vi "ParamsEntreferro.vi"(2 "paramsIn":variant=variant(cluster{"Componentes":cluster{"Pólo:":u16, "Amplitude:":dbl}[], "Num Polos":u16, "Folga Nominal":dbl, "Ruido":dbl} {"Componentes"=[], "Num Polos"=84, "Folga Nominal"=10.0, "Ruido"=1.0})) -> (16 "paramsOut":variant=variant(cluster{"Componentes":cluster{"Pólo:":u16, "Amplitude:":dbl}[], "Num Polos":u16, "Folga Nominal":dbl, "Ruido":dbl} {"Componentes"=[{"Pólo:"=2, "Amplitude:"=12.1}], "Num Polos"=20, "Folga Nominal"=10.0, "Ruido"=0.4}))   [LabVIEW 2017]
uses:
  Typedefs/Tipo_ComponenteSinalEntreferro.ctl
  Typedefs/Tipo_ParamsEntreferro.ctl
panel:
  in  "Ângulo (º)":dbl=0.4
  in  "Saturação":dbl=0.4
  in  "Ruído":dbl=0.4
  in  "Folga Nominal":dbl=10.0
  in  "N. Pólos":u16=20
  in  "Componentes":T1[](array[typedef])
  in  "Init":bool
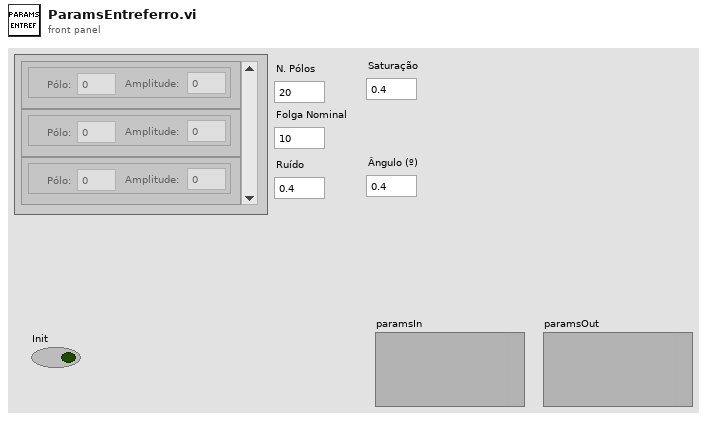
[diagram p1: front panel]
types:
  T1 = typedef "Tipo_ComponenteSinalEntreferro.ctl" = cluster{"Pólo:":u16, "Amplitude:":dbl}
  T2 = typedef "Tipo_ParamsEntreferro.ctl" = cluster{"Componentes":T1[], "Num Polos":u16, "Folga Nominal":dbl, "Ruido":dbl, "Saturacao":dbl, "Angulo":dbl}
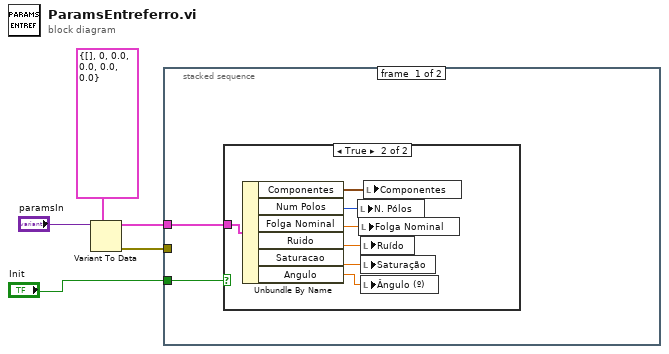
[diagram p0: block diagram]
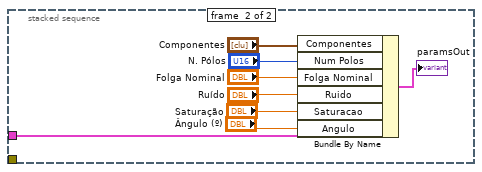
[diagram p3: hidden frame]
diagram:
  n1 = Variant To Data(type=T2 {"Componentes"=[], "Num Polos"=0, "Folga Nominal"=0.0, "Ruido"=0.0, "Saturacao"=0.0, "Angulo"=0.0}, Variant="paramsIn") -> (data=w4:T2, error out=w2:errorcluster)  [unwired: 1 in]
  n2 = stacked-sequence {
    tunnel: w4 -> [w7 w22]
    tunnel: "Init" -> [w6 _]
    tunnel: w2 -> [_ _]
    frame #0 {
      n3 = case shown="True" w6 {
        tunnel: w7 -> [_ w14]
        frame False {
        }
        frame True {
          n4 = Unbundle By Name(w14) -> ("Componentes"=w13:T1[], "Num Polos"=w12:u16, "Folga Nominal"=w11:dbl, "Ruido"=w10:dbl, "Saturacao"=w9:dbl, "Angulo"=w8:dbl)
          n5 = local write "N. Pólos"(w12) -> ()
          n6 = local write "Folga Nominal"(w11) -> ()
          n7 = local write "Ruído"(w10) -> ()
          n8 = local write "Saturação"(w9) -> ()
          n9 = local write "Ângulo (º)"(w8) -> ()
          n10 = local write "Componentes"(w13) -> ()
        }
      }
    }
    frame #1 {
      n11 = Bundle By Name(cluster=w22, "Componentes"="Componentes", "Num Polos"="N. Pólos", "Folga Nominal"="Folga Nominal", "Ruido"="Ruído", "Saturacao"="Saturação", "Angulo"="Ângulo (º)") -> (→"paramsOut":T2)
    }
  }
